vi "Shape Report to ROI SubVI.vi"(0 "Image In":T3, 2 "Shape Report":T2(array[cluster]) {"Score" format="%.2f"; "Centroid"."y" format="%.2f"; "Centroid"."x" format="%.2f"}, 3 "Error In":errorcluster) -> (7 "Image Out":T3, 9 "ROI Array Within Image":T1[](array[typedef]) {"Contours"."Type" items=["No Selection", "Point", "Line", "Rectangle", "Oval", "Polygon", "Freehand Region", "Annulus", "Unused2", "Unused3", "Broken Line", "Freehand Line", "Rotated Rectangle"]}, 10 "Error Out":errorcluster)   [LabVIEW 2014]
doc: "This subVI converts an array of shape reports into an array of ROI descriptions. It also takes in an image file, uses the shape report and ROI description to produce a duplicate image with the overlays of the ROI description."
uses:
  <vilib>/vision/Image Controls.llb/IMAQ Image.ctl
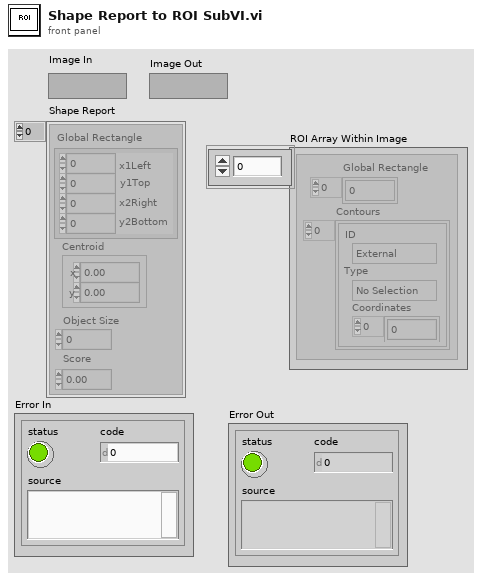
[diagram p1: front panel]
types:
  T1 = typedef "ROI Descriptor" = cluster{"Global Rectangle":i32[], "Contours":cluster{"ID":enum32{"External", "Internal"}, "Type":u32, "Coordinates":i32[]}[]}
  T2 = cluster{"Global Rectangle":cluster{"x1Left":i32, "y1Top":i32, "x2Right":i32, "y2Bottom":i32}, "Centroid":cluster{"x":sgl, "y":sgl}, "Object Size":u32, "Score":dbl}[]
  T3 = typedef "IMAQ Image.ctl" = refnum<image>
  T4 = cluster{"Global Rectangle":cluster{"x1Left":i32, "y1Top":i32, "x2Right":i32, "y2Bottom":i32}, "Centroid":cluster{"x":sgl, "y":sgl}, "Object Size":u32, "Score":dbl}
  T5 = cluster{"x1Left":i32, "y1Top":i32, "x2Right":i32, "y2Bottom":i32}
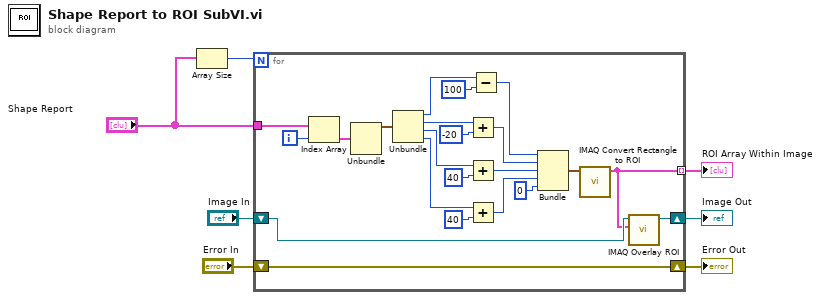
[diagram p0: block diagram]
diagram:
  n1 = Array Size(array="Shape Report") -> (size(s)=w1:i32)
  n2 = for {
    N: w1 -> [_]
    tunnel: "Shape Report" -> [w29]
    shift-right: [w12] -> w6
    shift-left: "Image In" -> [w11]
    tunnel: [w9] -> w5 mode=indexing
    shift-right: [w8] -> w3
    shift-left: "Error In" -> [w8]
    i -> [w10]
    n3 = Index Array(array=w29, index=w10) -> (element=w28:T4)
    n4 = Unbundle(w28) -> ("Global Rectangle"=w27:T5)  [unwired: 3 out]
    n5 = Unbundle(w27) -> ("x1Left"=w26:i32, "y1Top"=w22:i32, "x2Right"=w19:i32, "y2Bottom"=w17:i32)
    n6 = Add(x=w22, y=-20) -> (x+y=w23:i32)
    n7 = Add(x=w19, y=40) -> (x+y=w20:i32)
    n8 = Add(x=w17, y=40) -> (x+y=w15:i32)
    n9 = Subtract(x=w26, y=100) -> (x-y=w24:i32)
    n10 = Bundle(w24, w23, w20, w15, "y"=0) -> (w13:cluster{i32, i32, i32, i32, "y":i32})  [unwired: 1 in]
    n11 = call "IMAQ Convert Rectangle to ROI"("Rectangle"=w13) -> ("ROI Descriptor"=w9:T1)  [unwired: 8 in, 1 out]
    n12 = call "IMAQ Overlay ROI"("ROI Descriptor"=w9, "Image"=w11) -> ("Image Out"=w12:T3)  [unwired: 8 in, 1 out]
  }
  "Image Out" <- w6
  "ROI Array Within Image" <- w5
  "Error Out" <- w3
